vi "Final_v2._Sendvi.vi"() -> ()   [LabVIEW 2019]
uses:
  src/class/mqtt/mqttTypedef/mqttBroker.ctl
  src/class/mqtt/mqttTypedef/mqttConnectionFlags.ctl
  src/class/mqtt/mqttTypedef/mqttWillInformation.ctl
  src/class/mqtt/mqttConfigFunction.ctl
  src/class/mqtt/mqttTXqueue/mqttTXdataQueueFunction.ctl
  src/class/mqtt/mqttTXqueue/mqttRXsubscriptionEventFunction.ctl
  src/class/mqtt/mqttTypedef/mqttSubscribeCluster.ctl
  src/class/mqtt/mqttTypedef/mqttQOSlevel.ctl
  src/class/mqtt/mqtt.lvclass
panel:
  out "millisecond timer value":u32
  out "電暖爐 Flag":bool
  out "電扇 Flag":bool
  out "電燈 Flag":bool
  out "dis-success":bool
  out "Subscripts Data":string
  out "Subscripts Topic":string
  out "subscripts-status":bool
  out "Publish Data":string
  out "publish-status":bool
  out "Publish Topic":string
  in  "publish":bool
  in  "disconnect":bool
  in  "connect":bool
  out "MQTT Status":bool
  out "電暖爐":bool
  in  "電暖爐 手動開關":bool
  out "Temp L Flag":bool
  out "Temp H Flag":bool
  out "Door Flag":bool
  out "電扇":bool
  out "Boolean 73":bool
  out "Boolean 72":bool
  out "Boolean 71":bool
  out "Boolean 43":bool
  out "Boolean 70":bool
  out "Boolean 69":bool
  out "Boolean 68":bool
  out "Boolean 67":bool
  out "Boolean 66":bool
  out "Boolean 65":bool
  out "Boolean 64":bool
  out "Boolean 63":bool
  out "Boolean 62":bool
  out "Boolean 61":bool
  out "Boolean 60":bool
  out "Boolean 59":bool
  out "Boolean 58":bool
  out "Boolean 57":bool
  out "Boolean 56":bool
  out "Boolean 55":bool
  out "Boolean 54":bool
  out "Boolean 53":bool
  out "Boolean 52":bool
  out "Boolean 51":bool
  out "Boolean 50":bool
  out "Boolean 49":bool
  out "Boolean 48":bool
  out "Boolean 47":bool
  out "Boolean 46":bool
  out "Boolean 45":bool
  out "Boolean 44":bool
  out "Boolean 43":bool
  out "Boolean 42":bool
  out "Boolean 41":bool
  out "Boolean 40":bool
  out "Boolean 39":bool
  out "Boolean 38":bool
  out "Boolean 37":bool
  out "Boolean 36":bool
  out "Boolean 35":bool
  out "Boolean 34":bool
  out "Boolean 33":bool
  out "Boolean 32":bool
  out "Boolean 31":bool
  out "Boolean 30":bool
  out "Boolean 29":bool
  in  "電扇 手動開關":bool
  in  "Color Box":u32(colorbox)
  in  "電燈 手動開關":bool
  out "Table":string[][](table)
  in  "Stop Button":bool
  out "溫度過低":bool
  out "溫度過高":bool
  out "溫度下限(*C)":dbl
  out "溫度上限(*C)":dbl
  in  "溫度上下限":cluster{dbl, dbl}(slide) scale=0.0..40.0
  out "溫度表":dbl(slide) scale=0.0..40.0
  out "溫度(*C)":dbl format="%#.2g"
  out "開門":bool
  out "電燈":bool
  # "MQTT"
  # "MQTT-Status"
  # "Subscripts Topic"
  # "Publish-Status"
  # "Publish Topic"
  # "Subscripts-Status"
  # "Publish Data"
  # "Subscripts Data"
  # "溫度計"
  # "監控介面"
  # "現在時間"
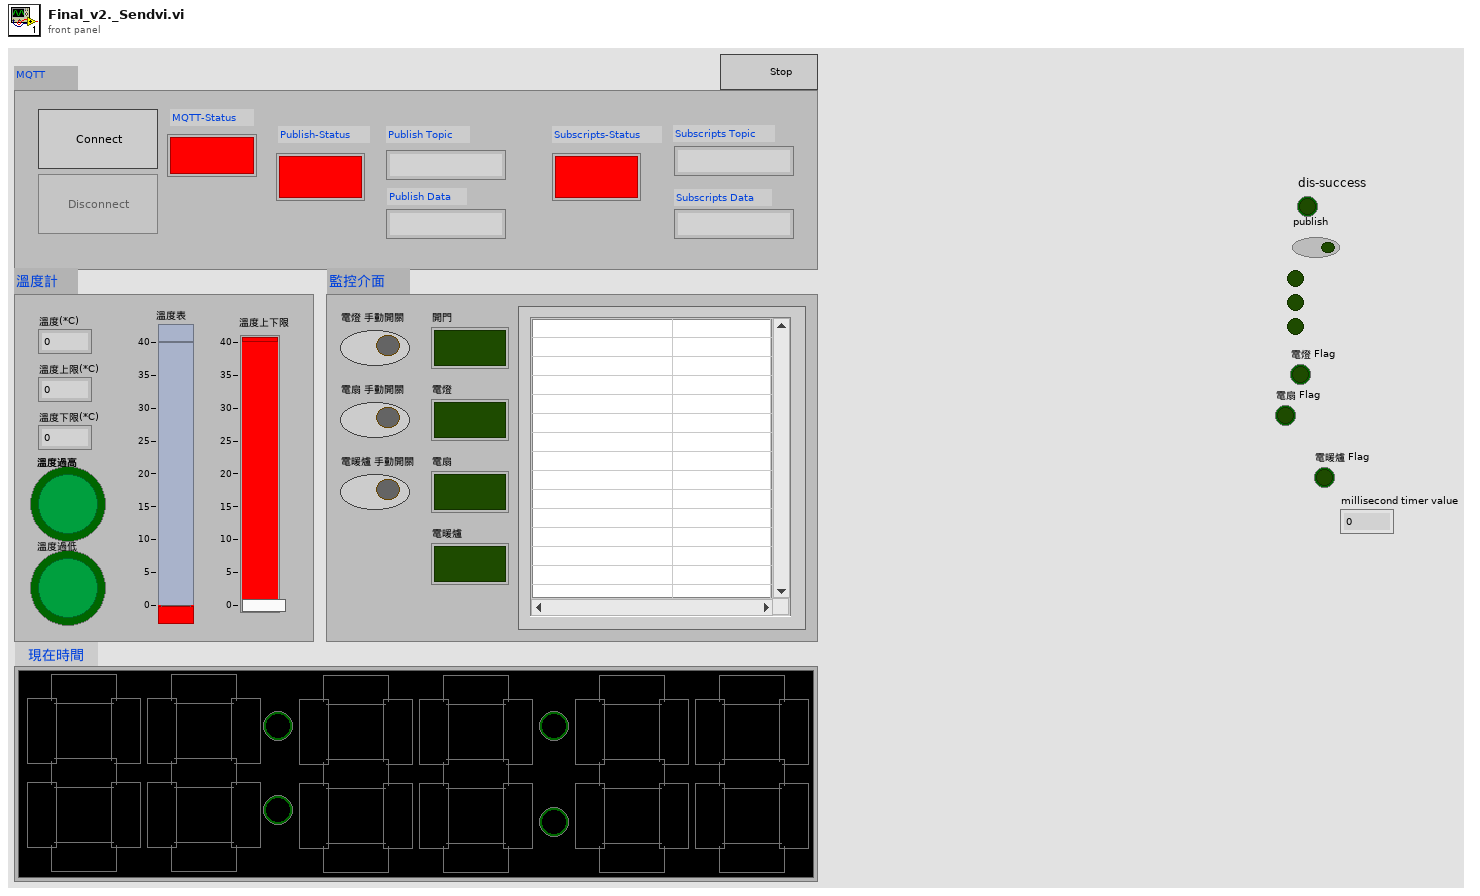
[diagram p1: front panel]
types:
  T1 = typedef "mqttRXsubscriptionEventFunction.ctl" = enum16{"init", "deinit", "getEventRef", "event"}
  T2 = typedef "mqttTXdataQueueFunction.ctl" = enum16{"init", "deinit", "getQueue", "enqueue"}
  T3 = typedef "mqtt.lvclass/mqttConfigFunction.ctl" = enum16{"init", "deinit", "set", "get"}
  T4 = typedef "mqttWillInformation.ctl" = cluster{"User Name":string, "Password":string}
  T5 = typedef "mqttConnectionFlags.ctl" = cluster{"reserved":bool, "clean session":bool, "will flag":bool, "willQOS":enum8{"At most once", "At least once", "Exactly once", "Reserved"}, "will retain":bool, "password":bool, "user name":bool}
  T6 = typedef "mqttBroker.ctl" = cluster{"address":string, "port":u16, "connTimeout":i32, "writeTimeout":i32, "readTimeout":i32, "subTimeout":i32}
  T7 = enum8{"Enabled", "Disabled", "Disabled and Grayed Out"}
  T8 = cluster{bool, bool, bool, bool, bool, bool, bool}[]
  T9 = cluster{bool, bool, bool, bool, bool, bool, bool}
  T10 = typedef "mqttSubscribeCluster.ctl" = cluster{"Topic":string, "QoS":T11}
  T11 = typedef "mqttQOSlevel.ctl" = enum8{"At most once", "At least once", "Exactly once", "Reserved"}
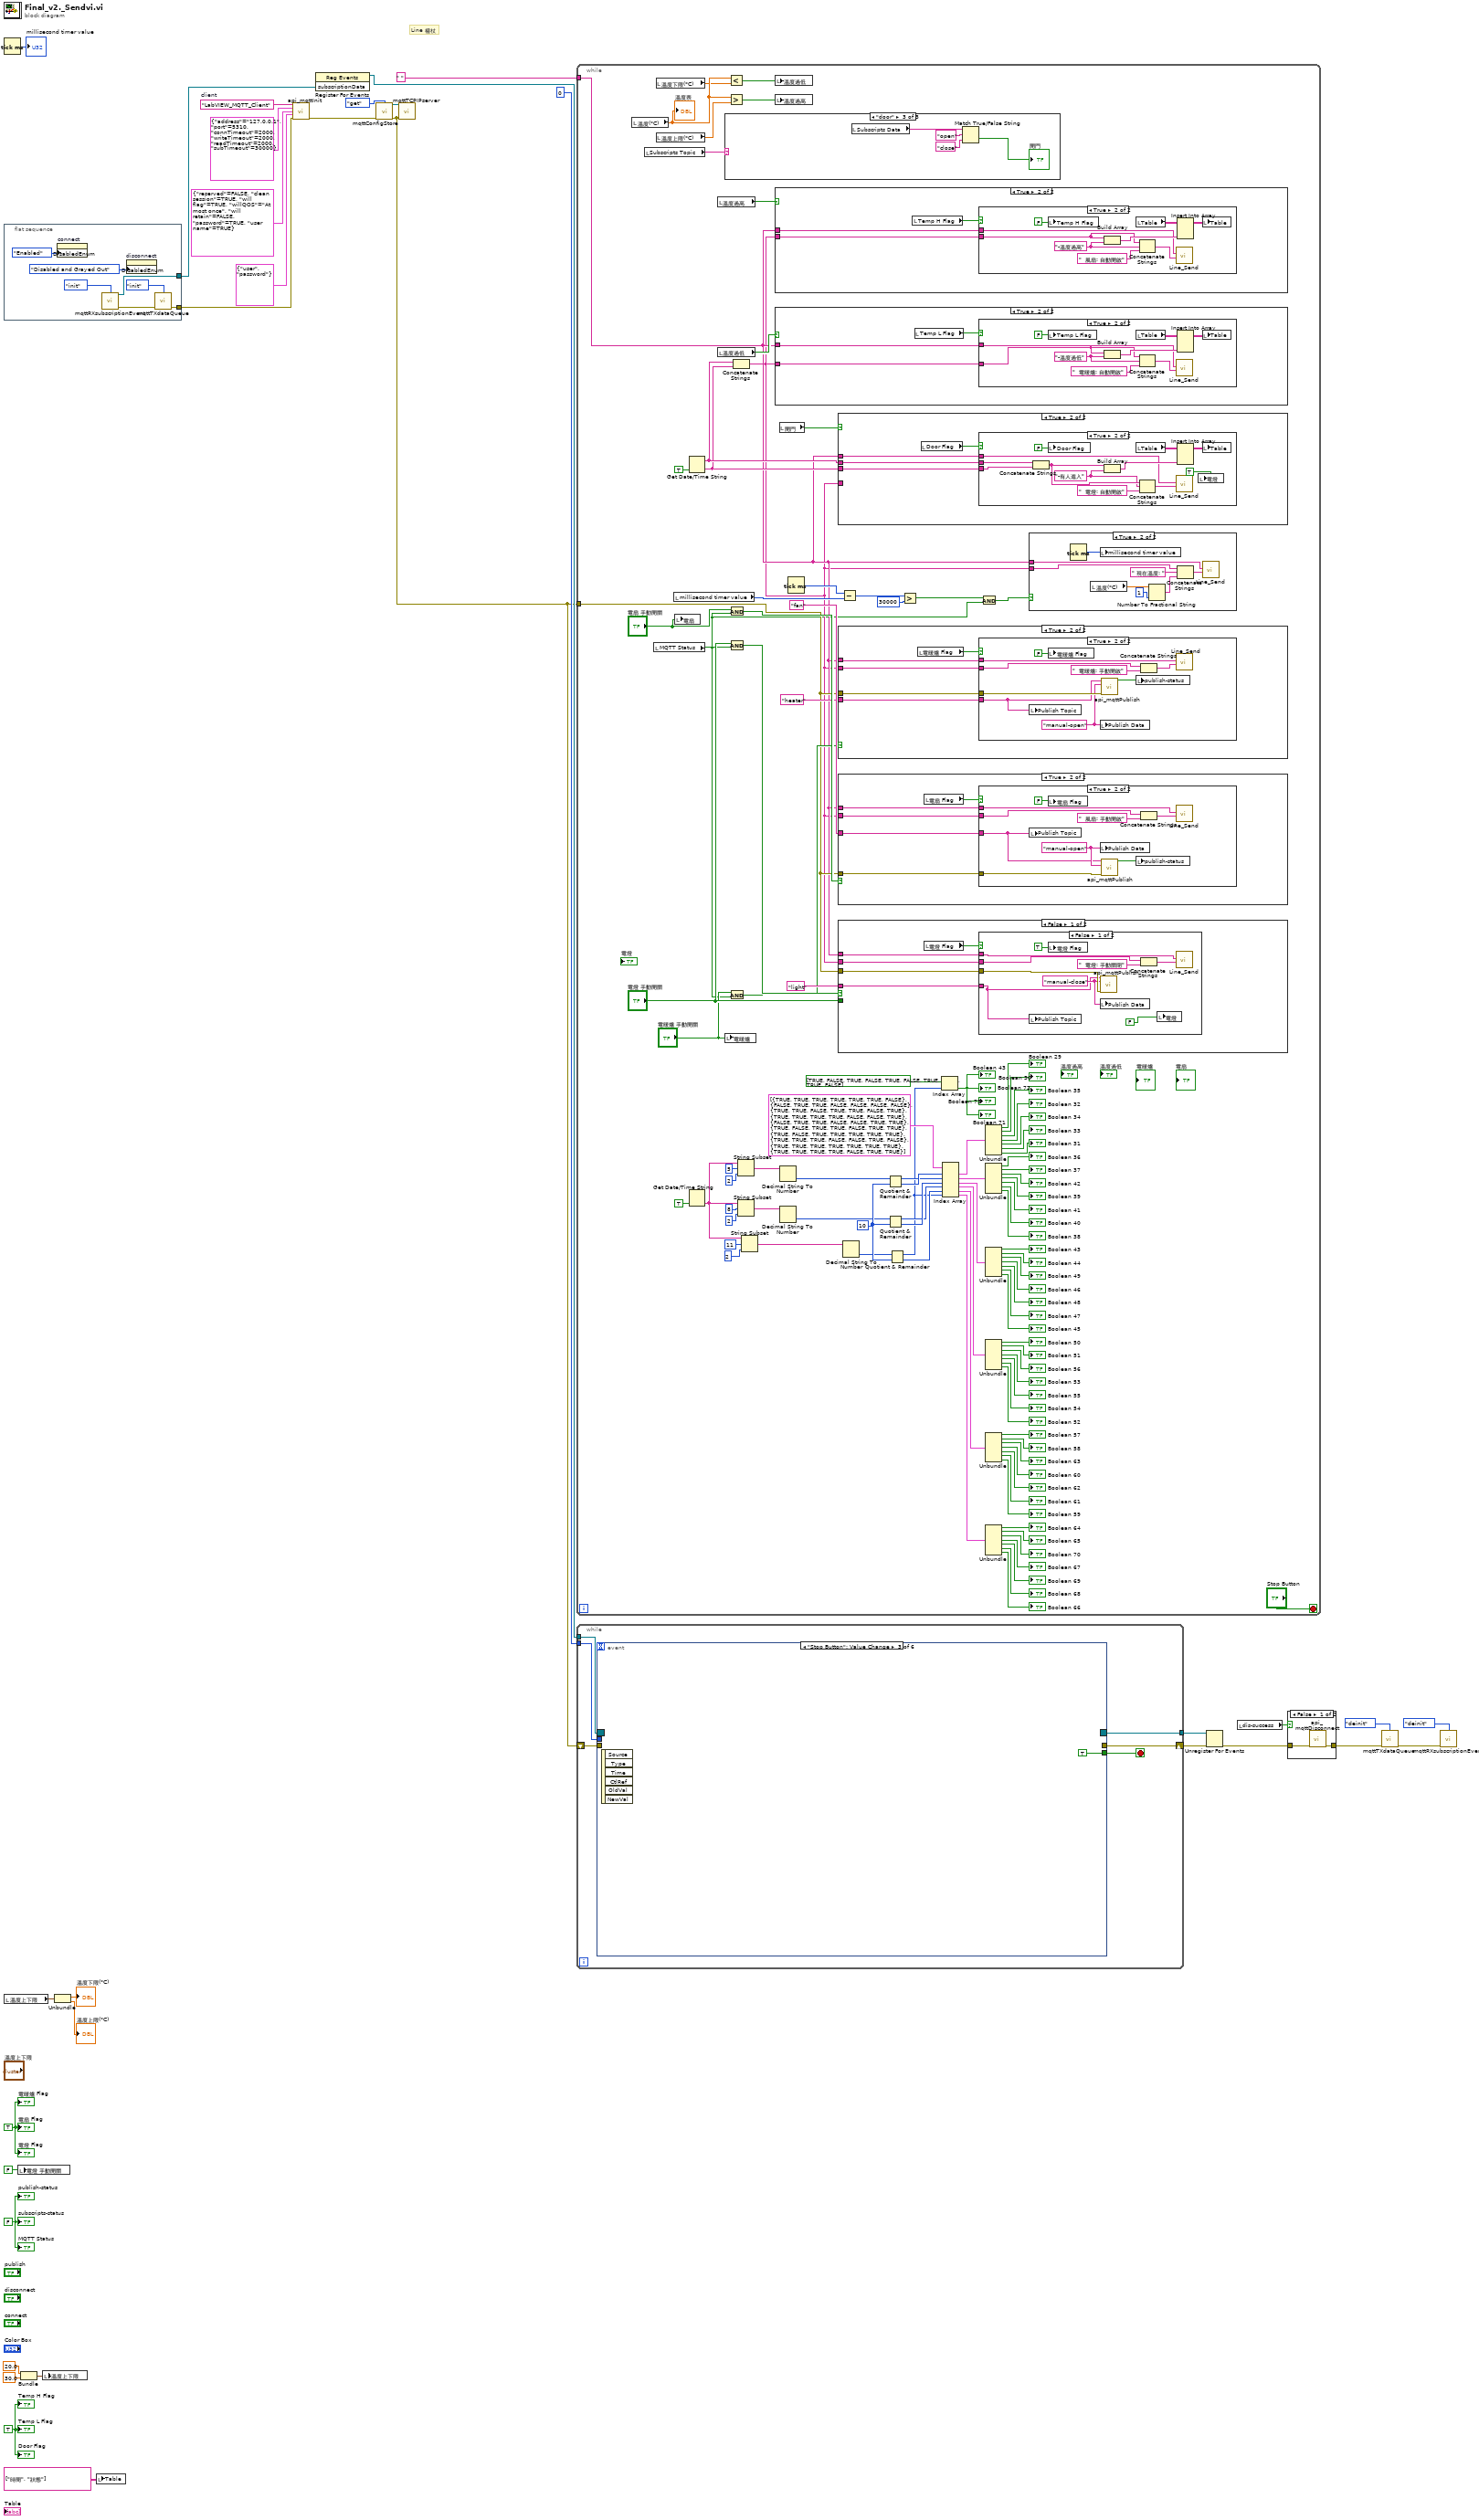
[diagram p0: block diagram]
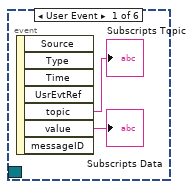
[diagram p3: hidden frame]
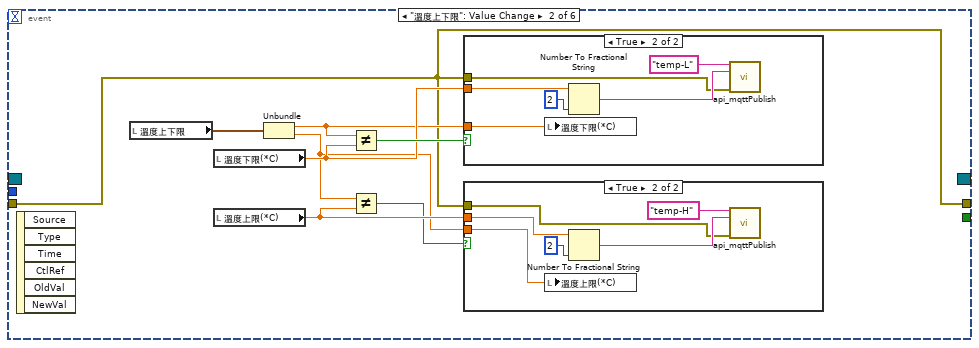
[diagram p4: hidden frame]
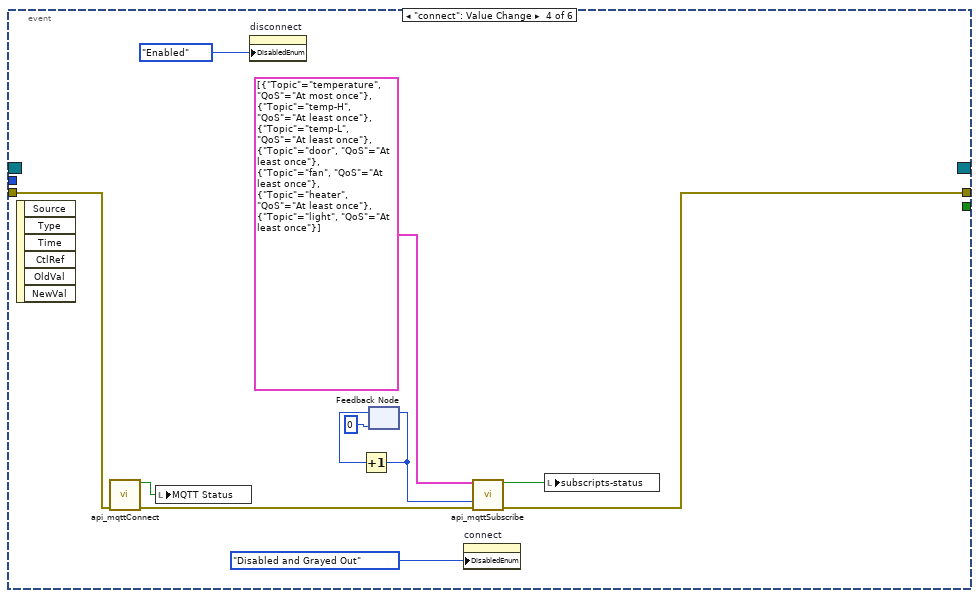
[diagram p7: hidden frame]
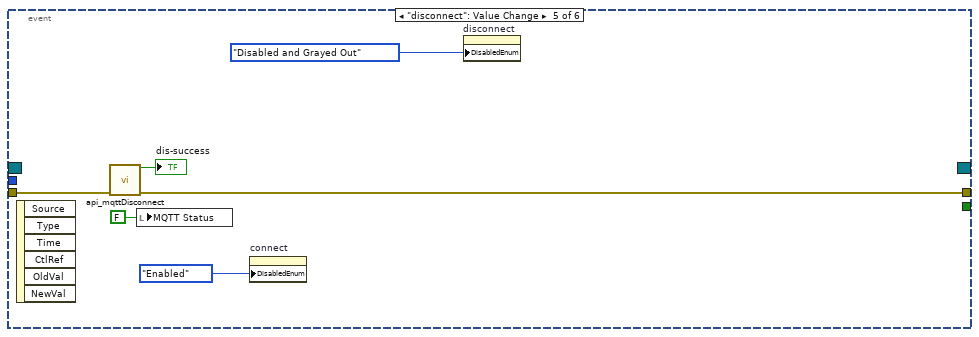
[diagram p8: hidden frame]
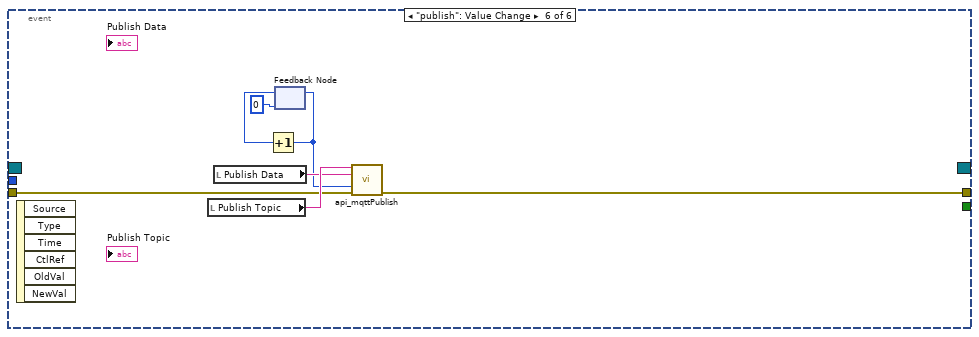
[diagram p9: hidden frame]
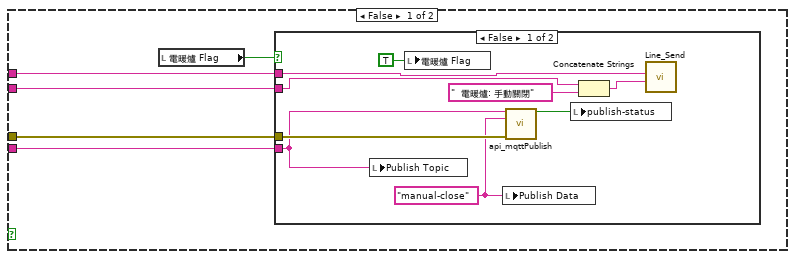
[diagram p11: hidden frame]
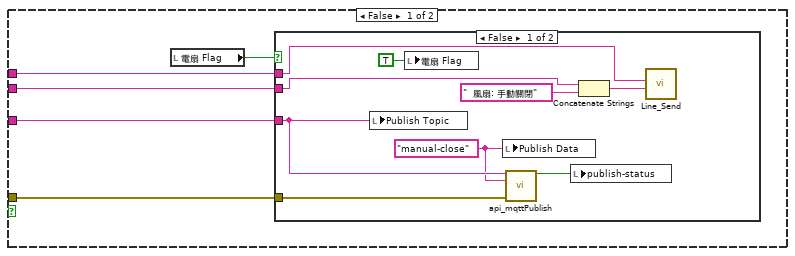
[diagram p14: hidden frame]
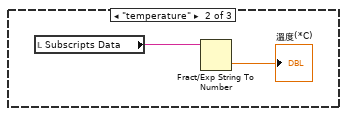
[diagram p18: hidden frame]
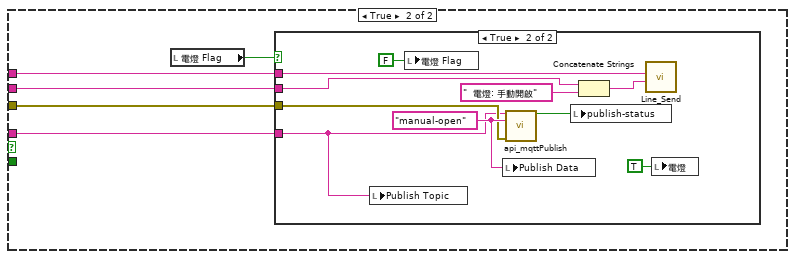
[diagram p20: hidden frame]
diagram:
  w6 = TRUE ("電燈 Flag")
  w25 = "LabVIEW_MQTT_Client"  # client
  w9 = FALSE ("MQTT Status")
  w32 = TRUE ("Door Flag")
  # "Line 權杖"
  n1 = Tick Count (ms)() -> (millisecond timer value=→"millisecond timer value":u32)
  n2 = flat-sequence {
    tunnel: [w39] -> w27
    tunnel: [w36] -> w20
    frame #0 {
      n3 = property on="connect" class="Bool"("DisabledEnum"=T7."Enabled" ("Disabled")) -> ()  [unwired: 2 in, 2 out]
      n4 = call "mqttRXsubscriptionEvent.vi"("function"=mqttRXsubscriptionEventFunction."init") -> ("subscriptionData"=w36:refnum<user-event>, "error out"=w38:errorcluster)  [unwired: 13 in]
      n5 = property on="disconnect" class="Bool (strict)"("DisabledEnum"=T7."Disabled and Grayed Out" ("Disabled")) -> ()  [unwired: 2 in, 2 out]
      n6 = call "mqttTXdataQueue.vi"("function"=mqttTXdataQueueFunction."init", "error in (no error)"=w38) -> ("error out"=w39:errorcluster)  [unwired: 12 in, 1 out]
    }
  }
  n7 = local read "溫度上下限"() -> (w3:cluster{dbl, dbl})
  n8 = local write "電燈 手動開關"(FALSE ("電燈 手動開關")) -> ()
  n9 = Bundle(20.0, 30.0) -> (w31:cluster{dbl, dbl})  [unwired: 1 in]
  n10 = local write "溫度上下限"(w31) -> ()
  n11 = Unbundle(w3) -> (→"溫度下限(*C)":dbl, →"溫度上限(*C)":dbl)
  n12 = local write "Table"(string[][] [["時間", "狀態"]]) -> ()
  n13 = call "api_mqttInit.vi"("client"=w25, "broker"=T6 {"address"="127.0.0.1", "port"=5310, "connTimeout"=2000, "writeTimeout"=2000, "readTimeout"=2000, "subTimeout"=30000}, "connFlags"=T5 {"reserved"=FALSE, "clean session"=TRUE, "will flag"=TRUE, "willQOS"=enum."At most once", "will retain"=FALSE, "password"=TRUE, "user name"=TRUE}, "User Info"=T4 {"User Name"="user", "Password"="password"}, "error in (no error)"=w27) -> ("error out"=w26:errorcluster)  [unwired: 10 in]
  n14 = register-events(w20) -> (reference out=w19:refnum<event-registration>)  [unwired: 2 in, 1 out]
  n15 = call "mqttConfigStore.vi"("function"=mqttConfigFunction."get", "error in (no error)"=w26) -> ("mqtt.lvclass out"=w21:refnum<class "mqtt.lvclass">, "error out"=w8:errorcluster)  [unwired: 12 in]
  n16 = call "mqttTCPIPserver.vi"("mqtt.lvclass"=w21, "error in (no error)"=w8) -> ()  [unwired: 12 in, 2 out]
  n17 = while {
    tunnel: w8 -> [w60]
    tunnel: " " -> [w45]
    stop <- "Stop Button" stop-if-true
    w85 = 10 ("y")
    n18 = local read "溫度(*C)"() -> (w59:dbl)
    "溫度表" <- w59
    n19 = local read "Subscripts Topic"() -> (w70:string)
    n20 = local read "MQTT Status"() -> (w41:bool)
    n21 = local read "溫度下限(*C)"() -> (w57:dbl)
    n22 = local read "溫度上限(*C)"() -> (w58:dbl)
    n23 = local read "millisecond timer value"() -> (w48:u32)
    n24 = local write "電扇"("電扇 手動開關") -> ()
    n25 = Get Date/Time String(want seconds? (F)=TRUE) -> (date string=w54:string, time string=w53:string)  [unwired: 2 in]
    n26 = Get Date/Time String(want seconds? (F)=TRUE) -> (time string=w76:string)  [unwired: 2 in, 1 out]
    n27 = local read "溫度過高"() -> (w51:bool)
    n28 = local read "溫度過低"() -> (w50:bool)
    n29 = case shown="\"door\"" w70 {
      frame "None", Default {
      }
      frame "temperature" {
        n30 = local read "Subscripts Data"() -> (w210:string)
        n31 = Fract/Exp String To Number(string=w210) -> (number=→"溫度(*C)":dbl)  [unwired: 3 in, 1 out]
      }
      frame "door" {
        n32 = local read "Subscripts Data"() -> (w214:string)
        n33 = Match True/False String(2:"close" ("false string"), 3:"open", 4:w214) -> (0:→"開門":bool)  [unwired: 1 out]
      }
    }
    n34 = local write "電暖爐"("電暖爐 手動開關") -> ()
    n35 = Less?(x=w59, y=w57) -> (x < y?=w55:bool)
    n36 = Greater?(x=w59, y=w58) -> (0:w56:bool)
    n37 = And(x="電扇 手動開關", y=w41) -> (x .and. y?=w67:bool)
    n38 = And(x="電暖爐 手動開關", y=w41) -> (x .and. y?=w63:bool)
    n39 = Compound Arithmetic op=AND("電燈 手動開關", w41) -> (w69:bool)
    n40 = Concatenate Strings(w54, w53) -> (w44:string)
    n41 = String Subset(string=w76, offset (0)=5, length (rest)=2 ("length (rest)")) -> (substring=w95:string)
    n42 = String Subset(string=w76, offset (0)=8, length (rest)=2 ("length (rest)")) -> (substring=w94:string)
    n43 = String Subset(string=w76, offset (0)=11, length (rest)=2 ("length (rest)")) -> (substring=w87:string)
    n44 = local write "溫度過低"(w55) -> ()
    n45 = local write "溫度過高"(w56) -> ()
    n46 = case shown="True" w51 {
      tunnel: w45 -> [w266 w274]
      tunnel: w44 -> [w265 w273]
      frame False {
        n47 = local read "Temp H Flag"() -> (w264:bool)
        n48 = case shown="False" w264 {
          tunnel: w266 -> [w268 _]
          tunnel: w265 -> [w267 _]
          frame False {
            n49 = local write "Temp H Flag"(TRUE) -> ()
            n50 = Concatenate Strings(w267, "  風扇: 自動關閉" ("string")) -> (w270:string)
            n51 = call "Line_Send.vi"("message"=w270, "Key"=w268) -> ()  [unwired: 10 in]
          }
          frame True {
          }
        }
      }
      frame True {
        n52 = local read "Temp H Flag"() -> (w272:bool)
        n53 = case shown="True" w272 {
          tunnel: w274 -> [_ w277]
          tunnel: w273 -> [_ w275]
          frame False {
          }
          frame True {
            w276 = "-溫度過高"
            n54 = local write "Temp H Flag"(FALSE ("Temp H Flag")) -> ()
            n55 = Build Array(w275, w276) -> (w282:string[])
            n56 = local read "Table"() -> (w283:string[][])
            n57 = Concatenate Strings(w275, w276, "  風扇: 自動開啟" ("string")) -> (w279:string)
            n58 = call "Line_Send.vi"("message"=w279, "Key"=w277) -> ()  [unwired: 10 in]
            n59 = Insert Into Array(array=w283, new element=w282) -> (w281:string[][])  [unwired: 2 in]
            n60 = local write "Table"(w281) -> ()
          }
        }
      }
    }
    n61 = case shown="True" w50 {
      tunnel: w45 -> [w245 w254]
      tunnel: w44 -> [w246 w253]
      frame False {
        n62 = local read "Temp L Flag"() -> (w244:bool)
        n63 = case shown="False" w244 {
          tunnel: w246 -> [w248 _]
          tunnel: w245 -> [w247 _]
          frame False {
            n64 = local write "Temp L Flag"(TRUE ("Temp L Flag")) -> ()
            n65 = Concatenate Strings(w248, "  電暖爐: 自動關閉" ("string")) -> (w250:string)
            n66 = call "Line_Send.vi"("message"=w250, "Key"=w247) -> ()  [unwired: 10 in]
          }
          frame True {
          }
        }
      }
      frame True {
        n67 = local read "Temp L Flag"() -> (w252:bool)
        n68 = case shown="True" w252 {
          tunnel: w254 -> [_ w257]
          tunnel: w253 -> [_ w256]
          frame False {
          }
          frame True {
            w255 = "-溫度過低"
            n69 = local write "Temp L Flag"(FALSE ("Temp L Flag")) -> ()
            n70 = Build Array(w256, w255) -> (w262:string[])
            n71 = local read "Table"() -> (w261:string[][])
            n72 = Concatenate Strings(w256, w255, "  電暖爐: 自動開啟" ("string")) -> (w259:string)
            n73 = call "Line_Send.vi"("message"=w259, "Key"=w257) -> ()  [unwired: 10 in]
            n74 = Insert Into Array(array=w261, new element=w262) -> (w260:string[][])  [unwired: 2 in]
            n75 = local write "Table"(w260) -> ()
          }
        }
      }
    }
    n76 = local read "開門"() -> (w52:bool)
    n77 = Decimal String To Number(string=w95) -> (number=w86:i32)  [unwired: 2 in, 1 out]
    n78 = Decimal String To Number(string=w94) -> (number=w84:i32)  [unwired: 2 in, 1 out]
    n79 = Tick Count (ms)() -> (millisecond timer value=w49:u32)
    n80 = case shown="True" w52 {
      tunnel: w54 -> [_ w291]
      tunnel: w53 -> [_ w290]
      tunnel: w45 -> [w285 w289]
      tunnel: w44 -> [w286 _]
      frame False {
        n81 = local read "Door Flag"() -> (w284:bool)
        n82 = case shown="False" w284 {
          tunnel: w286 -> [_ _]
          tunnel: w285 -> [_ _]
          frame False {
            n83 = local write "Door Flag"(TRUE ("Door Flag")) -> ()
          }
          frame True {
          }
        }
      }
      frame True {
        n84 = local read "Door Flag"() -> (w288:bool)
        n85 = case shown="True" w288 {
          tunnel: w291 -> [_ w303]
          tunnel: w290 -> [_ w302]
          tunnel: w289 -> [_ w297]
          frame False {
          }
          frame True {
            w294 = "-有人進入"
            n86 = Concatenate Strings(w303, w302) -> (w295:string)
            n87 = local write "Door Flag"(FALSE ("Door Flag")) -> ()
            n88 = Build Array(w295, w294) -> (w301:string[])
            n89 = local read "Table"() -> (w299:string[][])
            n90 = Concatenate Strings(w295, w294, "  電燈: 自動開啟" ("string")) -> (w296:string)
            n91 = call "Line_Send.vi"("message"=w296, "Key"=w297) -> ()  [unwired: 10 in]
            n92 = Insert Into Array(array=w299, new element=w301) -> (w298:string[][])  [unwired: 2 in]
            n93 = local write "電燈"(TRUE ("電燈")) -> ()
            n94 = local write "Table"(w298) -> ()
          }
        }
      }
    }
    n95 = case shown="True" w63 {
      tunnel: "heater" -> [w155 w169]
      tunnel: w60 -> [w156 w170]
      tunnel: w45 -> [w154 w168]
      tunnel: w44 -> [w153 w167]
      frame False {
        n96 = local read "電暖爐 Flag"() -> (w157:bool)
        n97 = case shown="False" w157 {
          tunnel: w156 -> [w165 _]
          tunnel: w155 -> [w160 _]
          tunnel: w154 -> [w161 _]
          tunnel: w153 -> [w159 _]
          frame False {
            w158 = "manual-close"
            n98 = local write "Publish Topic"(w160) -> ()
            n99 = local write "電暖爐 Flag"(TRUE ("電暖爐 Flag")) -> ()
            n100 = local write "Publish Data"(w158) -> ()
            n101 = call "api_mqttPublish.vi"("topic"=w160, "value"=w158, "error in (no error)"=w165) -> ("success"=w164:bool)  [unwired: 11 in, 1 out]
            n102 = local write "publish-status"(w164) -> ()
            n103 = Concatenate Strings(w159, "  電暖爐: 手動關閉" ("string")) -> (w163:string)
            n104 = call "Line_Send.vi"("message"=w163, "Key"=w161) -> ()  [unwired: 10 in]
          }
          frame True {
          }
        }
      }
      frame True {
        n105 = local read "電暖爐 Flag"() -> (w171:bool)
        n106 = case shown="True" w171 {
          tunnel: w170 -> [_ w180]
          tunnel: w169 -> [_ w173]
          tunnel: w168 -> [_ w176]
          tunnel: w167 -> [_ w175]
          frame False {
          }
          frame True {
            w174 = "manual-open"
            n107 = local write "Publish Topic"(w173) -> ()
            n108 = local write "電暖爐 Flag"(FALSE ("電暖爐 Flag")) -> ()
            n109 = local write "Publish Data"(w174) -> ()
            n110 = call "api_mqttPublish.vi"("topic"=w173, "value"=w174, "error in (no error)"=w180) -> ("success"=w178:bool)  [unwired: 11 in, 1 out]
            n111 = local write "publish-status"(w178) -> ()
            n112 = Concatenate Strings(w175, "  電暖爐: 手動開啟" ("string")) -> (w177:string)
            n113 = call "Line_Send.vi"("message"=w177, "Key"=w176) -> ()  [unwired: 10 in]
          }
        }
      }
    }
    n114 = case shown="True" w67 {
      tunnel: w60 -> [w183 w198]
      tunnel: "fan" -> [w184 w197]
      tunnel: w44 -> [w181 w196]
      tunnel: w45 -> [w182 w195]
      frame False {
        n115 = local read "電扇 Flag"() -> (w185:bool)
        n116 = case shown="False" w185 {
          tunnel: w184 -> [w191 _]
          tunnel: w183 -> [w193 _]
          tunnel: w182 -> [w187 _]
          tunnel: w181 -> [w186 _]
          frame False {
            w190 = "manual-close"
            n117 = local write "Publish Topic"(w191) -> ()
            n118 = local write "電扇 Flag"(TRUE ("電扇 Flag")) -> ()
            n119 = local write "Publish Data"(w190) -> ()
            n120 = call "api_mqttPublish.vi"("topic"=w191, "value"=w190, "error in (no error)"=w193) -> ("success"=w192:bool)  [unwired: 11 in, 1 out]
            n121 = local write "publish-status"(w192) -> ()
            n122 = Concatenate Strings(w186, "  風扇: 手動關閉" ("string")) -> (w188:string)
            n123 = call "Line_Send.vi"("message"=w188, "Key"=w187) -> ()  [unwired: 10 in]
          }
          frame True {
          }
        }
      }
      frame True {
        n124 = local read "電扇 Flag"() -> (w199:bool)
        n125 = case shown="True" w199 {
          tunnel: w198 -> [_ w208]
          tunnel: w197 -> [_ w204]
          tunnel: w196 -> [_ w202]
          tunnel: w195 -> [_ w200]
          frame False {
          }
          frame True {
            w207 = "manual-open"
            n126 = local write "Publish Topic"(w204) -> ()
            n127 = local write "電扇 Flag"(FALSE) -> ()
            n128 = local write "Publish Data"(w207) -> ()
            n129 = call "api_mqttPublish.vi"("topic"=w204, "value"=w207, "error in (no error)"=w208) -> ("success"=w205:bool)  [unwired: 11 in, 1 out]
            n130 = local write "publish-status"(w205) -> ()
            n131 = Concatenate Strings(w202, "  風扇: 手動開啟" ("string")) -> (w201:string)
            n132 = call "Line_Send.vi"("message"=w201, "Key"=w200) -> ()  [unwired: 10 in]
          }
        }
      }
    }
    n133 = case shown="False" w69 {
      tunnel: w60 -> [w219 w233]
      tunnel: "電燈 手動開關" -> [_ _]
      tunnel: "light" ("Publish Topic") -> [w217 w231]
      tunnel: w44 -> [w216 w230]
      tunnel: w45 -> [w215 w229]
      frame False {
        n134 = local read "電燈 Flag"() -> (w218:bool)
        n135 = case shown="False" w218 {
          tunnel: w219 -> [w227 _]
          tunnel: w217 -> [w225 _]
          tunnel: w216 -> [w222 _]
          tunnel: w215 -> [w221 _]
          frame False {
            w226 = "manual-close" ("Publish Data")
            n136 = local write "Publish Topic"(w225) -> ()
            n137 = local write "電燈 Flag"(TRUE ("電燈 Flag")) -> ()
            n138 = call "api_mqttPublish.vi"("topic"=w225, "value"=w226, "error in (no error)"=w227) -> ()  [unwired: 11 in, 2 out]
            n139 = local write "Publish Data"(w226) -> ()
            n140 = Concatenate Strings(w222, "  電燈: 手動關閉" ("string")) -> (w224:string)
            n141 = local write "電燈"(FALSE) -> ()
            n142 = call "Line_Send.vi"("message"=w224, "Key"=w221) -> ()  [unwired: 10 in]
          }
          frame True {
          }
        }
      }
      frame True {
        n143 = local read "電燈 Flag"() -> (w232:bool)
        n144 = case shown="True" w232 {
          tunnel: w233 -> [_ w242]
          tunnel: w231 -> [_ w239]
          tunnel: w230 -> [_ w236]
          tunnel: w229 -> [_ w235]
          frame False {
          }
          frame True {
            w243 = "manual-open" ("Publish Data")
            n145 = local write "Publish Topic"(w239) -> ()
            n146 = local write "電燈 Flag"(FALSE) -> ()
            n147 = local write "Publish Data"(w243) -> ()
            n148 = call "api_mqttPublish.vi"("topic"=w239, "value"=w243, "error in (no error)"=w242) -> ("success"=w241:bool)  [unwired: 11 in, 1 out]
            n149 = local write "publish-status"(w241) -> ()
            n150 = Concatenate Strings(w236, "  電燈: 手動開啟" ("string")) -> (w238:string)
            n151 = call "Line_Send.vi"("message"=w238, "Key"=w235) -> ()  [unwired: 10 in]
            n152 = local write "電燈"(TRUE ("電燈")) -> ()
          }
        }
      }
    }
    n153 = Subtract(x=w49, y=w48) -> (x-y=w47:u32)
    n154 = Decimal String To Number(string=w87) -> (number=w83:i32)  [unwired: 2 in, 1 out]
    n155 = Quotient & Remainder(x=w86, y=w85) -> (x-y*floor(x/y)=w81:i32, floor(x/y)=w82:i32)
    n156 = Quotient & Remainder(x=w84, y=w85) -> (x-y*floor(x/y)=w79:i32, floor(x/y)=w80:i32)
    n157 = Quotient & Remainder(x=w83, y=w85) -> (x-y*floor(x/y)=w75:i32, floor(x/y)=w78:i32)
    n158 = Greater?(x=w47, y=u32 30000) -> (0:w43:bool)
    n159 = Index Array(array=bool[] [TRUE, FALSE, TRUE, FALSE, TRUE, FALSE, TRUE, FALSE, TRUE, FALSE], index=w75) -> (element=→"Boolean 43" →"Boolean 71" →"Boolean 72" →"Boolean 73":bool)
    n160 = Index Array(array=T8 [{TRUE, TRUE, TRUE, TRUE, TRUE, TRUE, FALSE}, {FALSE, TRUE, TRUE, FALSE, FALSE, FALSE, FALSE}, {TRUE, TRUE, FALSE, TRUE, TRUE, FALSE, TRUE}, {TRUE, TRUE, TRUE, TRUE, FALSE, FALSE, TRUE}, {FALSE, TRUE, TRUE, FALSE, FALSE, TRUE, TRUE}, {TRUE, FALSE, TRUE, TRUE, FALSE, TRUE, TRUE}, {TRUE, FALSE, TRUE, TRUE, TRUE, TRUE, TRUE}, {TRUE, TRUE, TRUE, FALSE, FALSE, TRUE, FALSE}, {TRUE, TRUE, TRUE, TRUE, TRUE, TRUE, TRUE}, {TRUE, TRUE, TRUE, TRUE, FALSE, TRUE, TRUE}], index #1=w82, index #2=w81, index #3=w80, index #4=w79, index #5=w78, index #6=w75) -> (element #1=w143:T9, element #2=w142:T9, element #3=w141:T9, element #4=w140:T9, element #5=w139:T9, element #6=w138:T9)
    n161 = And(x=w43, y=w41) -> (x .and. y?=w42:bool)
    n162 = Unbundle(w143) -> (→"Boolean 29":bool, →"Boolean 30":bool, →"Boolean 35":bool, →"Boolean 32":bool, →"Boolean 34":bool, →"Boolean 33":bool, →"Boolean 31":bool)
    n163 = Unbundle(w142) -> (→"Boolean 36":bool, →"Boolean 37":bool, →"Boolean 42":bool, →"Boolean 39":bool, →"Boolean 41":bool, →"Boolean 40":bool, →"Boolean 38":bool)
    n164 = Unbundle(w141) -> (→"Boolean 43":bool, →"Boolean 44":bool, →"Boolean 49":bool, →"Boolean 46":bool, →"Boolean 48":bool, →"Boolean 47":bool, →"Boolean 45":bool)
    n165 = Unbundle(w140) -> (→"Boolean 50":bool, →"Boolean 51":bool, →"Boolean 56":bool, →"Boolean 53":bool, →"Boolean 55":bool, →"Boolean 54":bool, →"Boolean 52":bool)
    n166 = Unbundle(w139) -> (→"Boolean 57":bool, →"Boolean 58":bool, →"Boolean 63":bool, →"Boolean 60":bool, →"Boolean 62":bool, →"Boolean 61":bool, →"Boolean 59":bool)
    n167 = Unbundle(w138) -> (→"Boolean 64":bool, →"Boolean 65":bool, →"Boolean 70":bool, →"Boolean 67":bool, →"Boolean 69":bool, →"Boolean 68":bool, →"Boolean 66":bool)
    n168 = case shown="True" w42 {
      tunnel: w45 -> [_ w150]
      tunnel: w44 -> [_ w148]
      frame False {
      }
      frame True {
        n169 = Tick Count (ms)() -> (millisecond timer value=w145:u32)
        n170 = local read "溫度(*C)"() -> (w152:dbl)
        n171 = local write "millisecond timer value"(w145) -> ()
        n172 = Number To Fractional String(number=w152, precision (6)=i16 1) -> (F-format string=w146:string)  [unwired: 2 in]
        n173 = Concatenate Strings(w148, " 現在溫度: " ("string"), w146) -> (w149:string)
        n174 = call "Line_Send.vi"("message"=w149, "Key"=w150) -> ()  [unwired: 10 in]
      }
    }
  }
  n175 = while {
    tunnel: w19 -> [w306]
    shift-right: [w307] -> w13
    shift-left: w8 -> [w308]
    tunnel: [w305] -> w12
    tunnel: 0 -> [w304]
    stop <- w309 stop-if-true
    n176 = event shown="[2] \"Stop Button\": Value Change" {
      selector: w306 -> [_ _ _ _ _ _]
      dyn-events: [_ _ _ _ _ _] -> w305
      timeout: _ -> [_ _ _ _ _ _]
      tunnel: [_ _ TRUE _ _ _] -> w309
      tunnel: w308 -> [_ w312 _ w343 w349 w351]
      tunnel: [_ w312 _ w337 w347 w350] -> w307
      tunnel: w304 -> [_ _ _ _ _ _]
      event User Event {
        n177 = event-data() -> ("topic"=→"Subscripts Topic":string, "value"=→"Subscripts Data":string)  [unwired: 1 in, 5 out]
      }
      event "溫度上下限": Value Change {
        n178 = event-data() -> ()  [unwired: 1 in, 6 out]
        n179 = local read "溫度上下限"() -> (w319:cluster{dbl, dbl})
        n180 = local read "溫度下限(*C)"() -> (w317:dbl)
        n181 = local read "溫度上限(*C)"() -> (w315:dbl)
        n182 = Unbundle(w319) -> (w316:dbl, w313:dbl)
        n183 = Not Equal?(x=w316, y=w317) -> (x != y?=w318:bool)
        n184 = Not Equal?(x=w313, y=w315) -> (x != y?=w314:bool)
        n185 = case shown="True" w318 {
          tunnel: w317 -> [_ w328]
          tunnel: w316 -> [_ w327]
          tunnel: w312 -> [_ w326]
          frame False {
          }
          frame True {
            n186 = local write "溫度下限(*C)"(w327) -> ()
            n187 = Number To Fractional String(number=w328, precision (6)=i16 2) -> (F-format string=w331:string)  [unwired: 2 in]
            n188 = call "api_mqttPublish.vi"("topic"="temp-L", "value"=w331, "error in (no error)"=w326) -> ()  [unwired: 11 in, 2 out]
          }
        }
        n189 = case shown="True" w314 {
          tunnel: w315 -> [_ w322]
          tunnel: w313 -> [_ w321]
          tunnel: w312 -> [_ w320]
          frame False {
          }
          frame True {
            n190 = local write "溫度上限(*C)"(w321) -> ()
            n191 = Number To Fractional String(number=w322, precision (6)=i16 2) -> (F-format string=w323:string)  [unwired: 2 in]
            n192 = call "api_mqttPublish.vi"("topic"="temp-H", "value"=w323, "error in (no error)"=w320) -> ()  [unwired: 11 in, 2 out]
          }
        }
      }
      event "Stop Button": Value Change {
        n193 = event-data() -> ()  [unwired: 1 in, 6 out]
      }
      event "connect": Value Change {
        n194 = event-data() -> ()  [unwired: 1 in, 6 out]
        n195 = call "api_mqttConnect.vi"("error in (no error)"=w343) -> ("success"=w336:bool, "error out"=w338:errorcluster)  [unwired: 11 in, 2 out]
        n196 = local write "MQTT Status"(w336) -> ()
        n197 = property on="disconnect" class="Bool (strict)"("DisabledEnum"=T7."Enabled" ("Disabled")) -> ()  [unwired: 2 in, 2 out]
        n198 = feedback #1(u16 0) -> (w341:u16)
        n199 = Increment(x=w341) -> (x+1=w340:u16)
        n200 = feedback-in #1(w340) -> ()
        n201 = property on="connect" class="Bool"("DisabledEnum"=T7."Disabled and Grayed Out" ("Disabled")) -> ()  [unwired: 2 in, 2 out]
        n202 = call "api_mqttSubscribe.vi"("subscriptionInfo"=T10[] [{"Topic"="temperature", "QoS"=enum."At most once"}, {"Topic"="temp-H", "QoS"=enum."At least once"}, {"Topic"="temp-L", "QoS"=enum."At least once"}, {"Topic"="door", "QoS"=enum."At least once"}, {"Topic"="fan", "QoS"=enum."At least once"}, {"Topic"="heater", "QoS"=enum."At least once"}, {"Topic"="light", "QoS"=enum."At least once"}], "messageID"=w340, "error in (no error)"=w338) -> ("success"=w333:bool, "error out"=w337:errorcluster)  [unwired: 11 in]
        n203 = local write "subscripts-status"(w333) -> ()
      }
      event "disconnect": Value Change {
        n204 = event-data() -> ()  [unwired: 1 in, 6 out]
        n205 = call "api_mqttDisconnect.vi"("error in (no error)"=w349) -> ("success"=→"dis-success":bool, "error out"=w347:errorcluster)  [unwired: 13 in]
        n206 = local write "MQTT Status"(FALSE) -> ()
        n207 = property on="connect" class="Bool"("DisabledEnum"=T7."Enabled" ("Disabled")) -> ()  [unwired: 2 in, 2 out]
        n208 = property on="disconnect" class="Bool (strict)"("DisabledEnum"=T7."Disabled and Grayed Out" ("Disabled")) -> ()  [unwired: 2 in, 2 out]
      }
      event "publish": Value Change {
        n209 = event-data() -> ()  [unwired: 1 in, 6 out]
        n210 = local read "Publish Topic"() -> (w356:string)
        n211 = local read "Publish Data"() -> (w355:string)
        n212 = feedback #2(u16 0) -> (w353:u16)
        n213 = Increment(x=w353) -> (x+1=w352:u16)
        n214 = feedback-in #2(w352) -> ()
        n215 = call "api_mqttPublish.vi"("topic"=w356, "value"=w355, "messageID"=w352, "error in (no error)"=w351) -> ("error out"=w350:errorcluster)  [unwired: 10 in, 1 out]
      }
    }
  }
  n216 = Unregister For Events(event registration refnum=w12, error in=w13) -> (error out=w14:errorcluster)
  n217 = local read "dis-success"() -> (w10:bool)
  n218 = case shown="False" w10 {
    tunnel: [w358 w359] -> w17
    tunnel: w14 -> [w357 w359]
    frame False {
      n219 = call "api_mqttDisconnect.vi"("error in (no error)"=w357) -> ("error out"=w358:errorcluster)  [unwired: 13 in, 1 out]
    }
    frame True {
    }
  }
  n220 = call "mqttTXdataQueue.vi"("function"=mqttTXdataQueueFunction."deinit", "error in (no error)"=w17) -> ("error out"=w15:errorcluster)  [unwired: 12 in, 1 out]
  n221 = call "mqttRXsubscriptionEvent.vi"("function"=mqttRXsubscriptionEventFunction."deinit", "error in (no error)"=w15) -> ()  [unwired: 12 in, 2 out]
  "Door Flag" <- w32
  "Temp H Flag" <- w32
  "Temp L Flag" <- w32
  "MQTT Status" <- w9
  "publish-status" <- w9
  "subscripts-status" <- w9
  "電燈 Flag" <- w6
  "電扇 Flag" <- w6
  "電暖爐 Flag" <- w6
